vi "sensor cmd battery voltage.vi"(10 "voltage":u16, 11 "device_handle":u32) -> (1 "function return":i32, 2 "voltage out":u16, 3 "device_handle out":u32)   [LabVIEW 2019, in "apdm.lvlib"]
doc: "APDM_EXPORT int apdm_sensor_cmd_battery_voltage(apdm_device_handle_t device_handle, uint16_t *voltage);"
uses:
  apdm.lvlib
  Lee Lab/CP FES Walking 2018/Code/Working/LabVIEW/apdm.dll
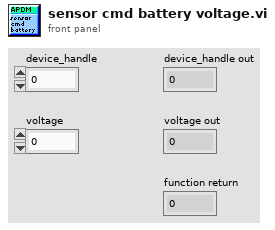
[diagram p1: front panel]
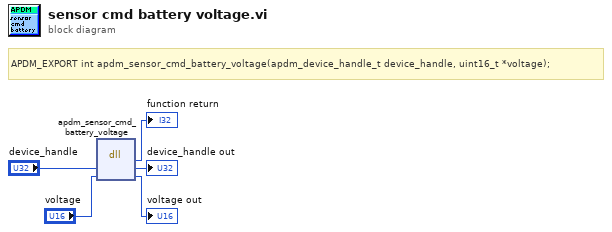
[diagram p0: block diagram]
diagram:
  # "APDM_EXPORT int apdm_sensor_cmd_battery_voltage(apdm_device_handle_t device_handle, uint16_t *voltage);"
  n1 = dll-call lib="C:/Users/jfalesi/Dropbox/Lee Lab/CP FES Walking 2018/Code/Working/LabVIEW/apdm.*" fn="apdm_sensor_cmd_battery_voltage"("device_handle"="device_handle", "voltage"="voltage") -> (→"function return":i32, "device_handle"=→"device_handle out":u32, "voltage"=→"voltage out":u16)  [unwired: 3 in, 2 out]
